vi "runtime_array.vi"() -> ()   [LabVIEW 2019]
uses:
  <vilib>/Analysis/Matrix/Datatypes/RealMatrix.ctl
  51b4a0fc-a318-4f67-9976-8ca54c98d554.vi
  <vilib>/Analysis/Matrix/Numeric/Conversions/Array To Matrix - RA.vi
  <vilib>/Analysis/Matrix/NI_Matrix.lvlib
panel:
  out "Real Matrix (Column Vector)":T1
  out "array with \nduplicates removed":dbl[](array[numeric])
  out "index of element":i32
  out "sorted array":dbl[](array[numeric])
  out "array (last n \nelements first)":dbl[](array[numeric])
  in  "Array":dbl[](array[numeric])
  out "initialized array":dbl[](array[numeric])
  out "appended array":dbl[](array[numeric])
  in  "element 5":dbl=5.0
  in  "element 4":dbl=4.0
  in  "element 3":dbl=3.0
  in  "element 2":dbl=2.0
  in  "element 1":dbl=1.0
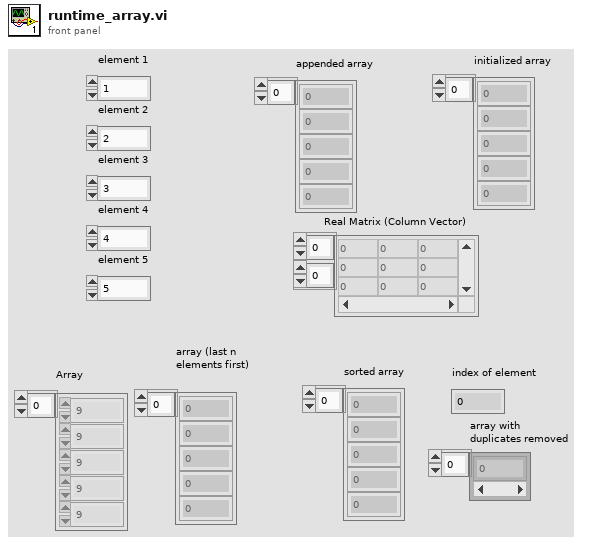
[diagram p1: front panel]
types:
  T1 = typedef "NI_Matrix.lvlib/RealMatrix.ctl" = dbl[][]
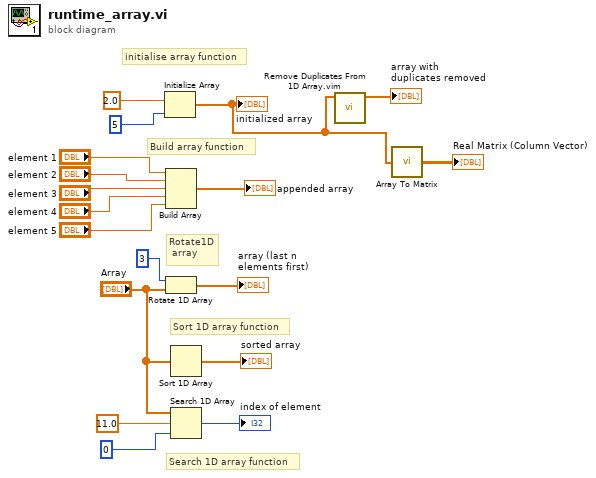
[diagram p0: block diagram]
diagram:
  # "initialise array function"
  # "Build array function"
  # "Rotate1D\n array"
  # "Sort 1D array function"
  # "Search 1D array function"
  n1 = Initialize Array(2.0 ("element"), 5 ("dimension size")) -> (w2:dbl[])
  "initialized array" <- w2
  n2 = Build Array("element 1", "element 2", "element 3", "element 4", "element 5") -> (→"appended array":dbl[])
  n3 = Rotate 1D Array(1:"Array", 2:3) -> (0:→"array (last n \nelements first)":dbl[])
  n4 = Sort 1D Array(array="Array") -> (sorted array=→"sorted array":dbl[])
  n5 = Search 1D Array(1D array="Array", element=11.0, start index (0)=0) -> (index of element=→"index of element":i32)
  n6 = call "Remove Duplicates From 1D Array.vim"("array"=w2) -> ("array with duplicates removed"=→"array with \nduplicates removed":dbl[])  [unwired: 10 in]
  n7 = call-poly <vilib>:"Array To Matrix.vi"("Real 1D Array"=w2) -> ("Real Matrix (Column Vector)"=→"Real Matrix (Column Vector)":T1)
